vi "Close.vi"(8 "error in (no error)":errorcluster, 11 "navX in":refnum<class "navX.lvclass">) -> (0 "error out":errorcluster)   [LabVIEW 2015, in "navX Library v3.lvlib" / "navX.lvclass"]
uses:
  navX.lvclass
  navX.lvclass/navX.ctl
  navX - Base/navX - Base.lvclass
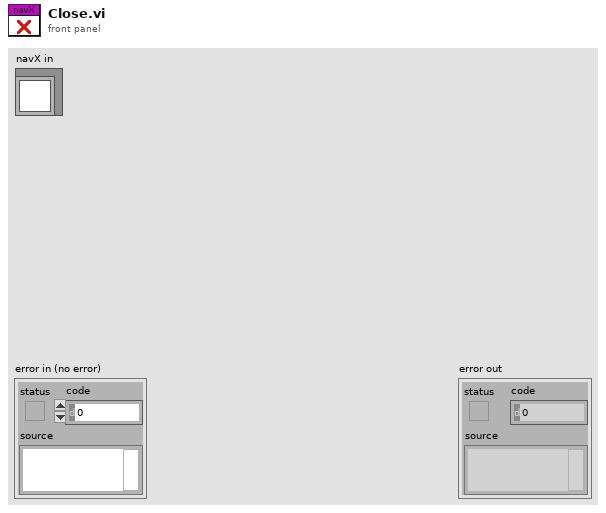
[diagram p1: front panel]
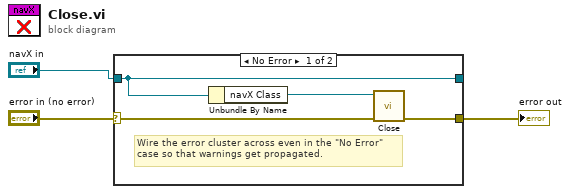
[diagram p0: block diagram]
diagram:
  n1 = case shown="No Error" "error in (no error)" {
    selector: "error in (no error)" -> [w5 w9]
    tunnel: [w4 w9] -> w2
    tunnel: [w7 w8] -> _
    tunnel: "navX in" -> [w7 w8]
    frame No Error {
      # "Wire the error cluster across even in the \"No Error\"\ncase so that warnings get propagated."
      n2 = Unbundle By Name(w7) -> ("navX Class"=w6:refnum<class "navX - Base.lvclass">)
      n3 = call-dynamic "Close.vi"("error in (no error)"=w5, "navX - Base in"=w6) -> ("error out"=w4:errorcluster)  [unwired: 8 in, 1 out]
    }
    frame Error {
    }
  }
  "error out" <- w2
